vi "panel_generate_stop_ui_event.vi"(8 "error in (no error)":errorcluster, 11 "panel in":refnum<class "panel.lvclass">) -> (0 "error out":errorcluster, 2 "stop_ui_ref":refnum<event-registration>, 3 "panel out":refnum<class "panel.lvclass">)   [LabVIEW 2015, in "panel.lvclass"]
uses:
  panel.lvclass
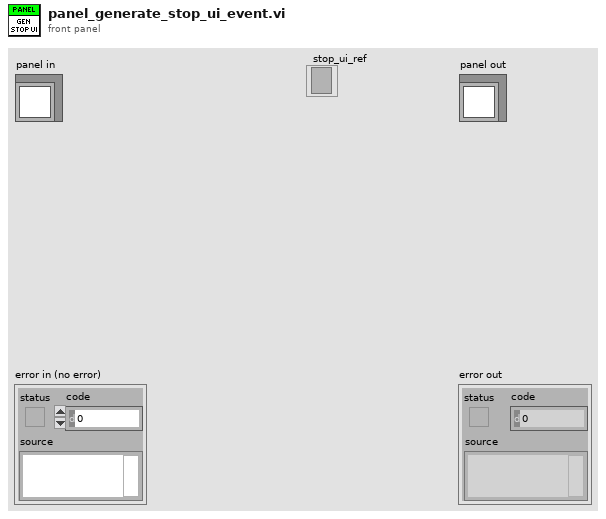
[diagram p1: front panel]
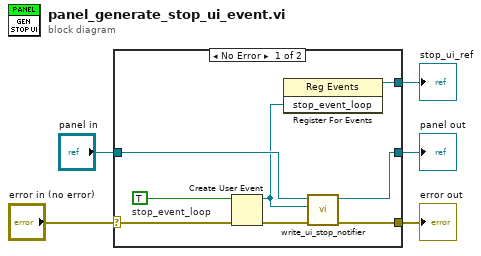
[diagram p0: block diagram]
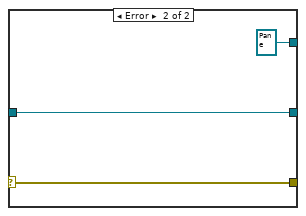
[diagram p2: hidden frame]
diagram:
  n1 = case shown="No Error" "error in (no error)" {
    selector: "error in (no error)" -> [w12 w16]
    tunnel: [w6 w16] -> w4
    tunnel: [w9 w15] -> w2
    tunnel: "panel in" -> [w10 w15]
    tunnel: [w7 refnum<event-registration> refnum ("Event Registration Refnum")] -> w1
    frame No Error {
      w13 = TRUE  # stop_event_loop
      n2 = Create User Event(user event datatype=w13, error in=w12) -> (user event=w8:refnum<user-event>, error out=w11:errorcluster)
      n3 = register-events(w8) -> (reference out=w7:refnum<event-registration>)  [unwired: 2 in, 1 out]
      n4 = call "write_ui_stop_notifier.vi"("error in (no error)"=w11, "stop_ui_notifier"=w8, "panel in"=w10) -> ("error out"=w6:errorcluster, "panel out"=w9:refnum<class "panel.lvclass">)  [unwired: 7 in]
    }
    frame Error {
    }
  }
  "error out" <- w4
  "panel out" <- w2
  "stop_ui_ref" <- w1
